vi "AIT 664 - Add Rx Message Port.vi"(0 "Item Ref in":T4 format="%.0x", 5 "Rx Message Port":T1, 11 "error in (no error)":errorcluster) -> (15 "error out":errorcluster)   [LabVIEW 2013, in "AIT 664 Custom Device.lvlib"]
doc: "Add Rx Message Port"
uses:
  AIT 664 Custom Device.lvlib
  <vilib>/NI Veristand/Custom Device API/Custom Device Item Ref.ctl
  Controls/664 - XML Rx Message Port.ctl
  Controls/664 - Sampling Type.ctl
  Controls/664 -Param.ctl
  <vilib>/NI Veristand/Custom Device API/Custom Device Channel.ctl
  <vilib>/NI Veristand/Custom Device API/Custom Device Channel Type.ctl
  Controls and Global/Global.vi
  <vilib>/NI Veristand/Custom Device API/Set Item Property (U32).vi
  <vilib>/NI Veristand/Custom Device API/Set Item Property (Variant).vi
  <vilib>/NI Veristand/Custom Device API/Set Item Property (String).vi
  <vilib>/NI Veristand/Custom Device API/Set Item Property (Boolean).vi
  <vilib>/NI Veristand/Custom Device API/Custom Device API.lvlib
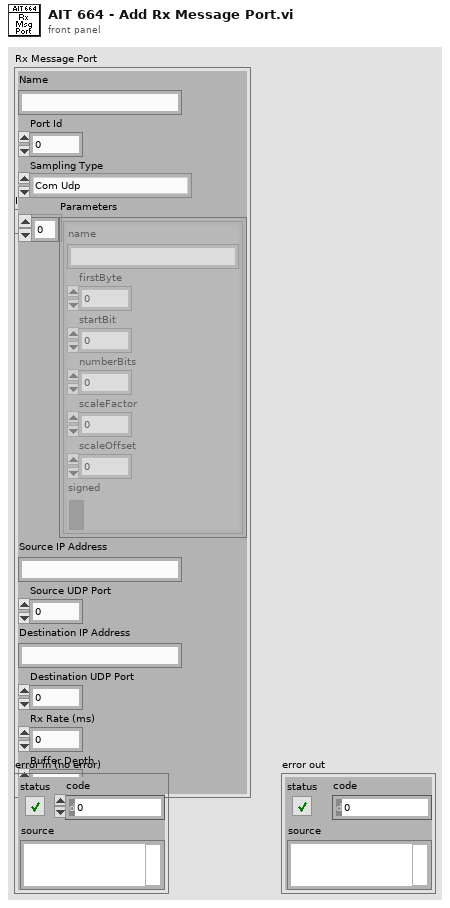
[diagram p1: front panel]
types:
  T1 = typedef "AIT 664 Custom Device.lvlib/664 - XML Rx Message Port.ctl" = cluster{"Name":string, "Port Id":u32, "Sampling Type":T2, "Parameters":T3[], "Source IP Address":string, "Source UDP Port":u32, "Destination IP Address":string, "Destination UDP Port":u32, "Rx Rate (ms)":u32, "Buffer Depth":u32}
  T2 = typedef "AIT 664 Custom Device.lvlib/664 - Sampling Type.ctl" = enum16{"Com Udp", "Com Udp Queuing", "Sap Udp", "Sap Ip", "Sap Mac", "Unknown"}
  T3 = typedef "AIT 664 Custom Device.lvlib/664 -Param.ctl" = cluster{"name":string, "firstByte":i32, "startBit":i32, "numberBits":i32, "scaleFactor":dbl, "scaleOffset":dbl, "signed":bool}
  T4 = typedef "Custom Device API.lvlib/Custom Device Item Ref.ctl" = u64
  T5 = typedef "Custom Device API.lvlib/Custom Device Channel Type.ctl" = enum16{"Input", "Output"}
  T6 = typedef "Custom Device API.lvlib/Custom Device Channel.ctl" = cluster{"Type":T5, "Units":string, "Default Value":dbl, "Faultable":bool, "Scalable":bool}
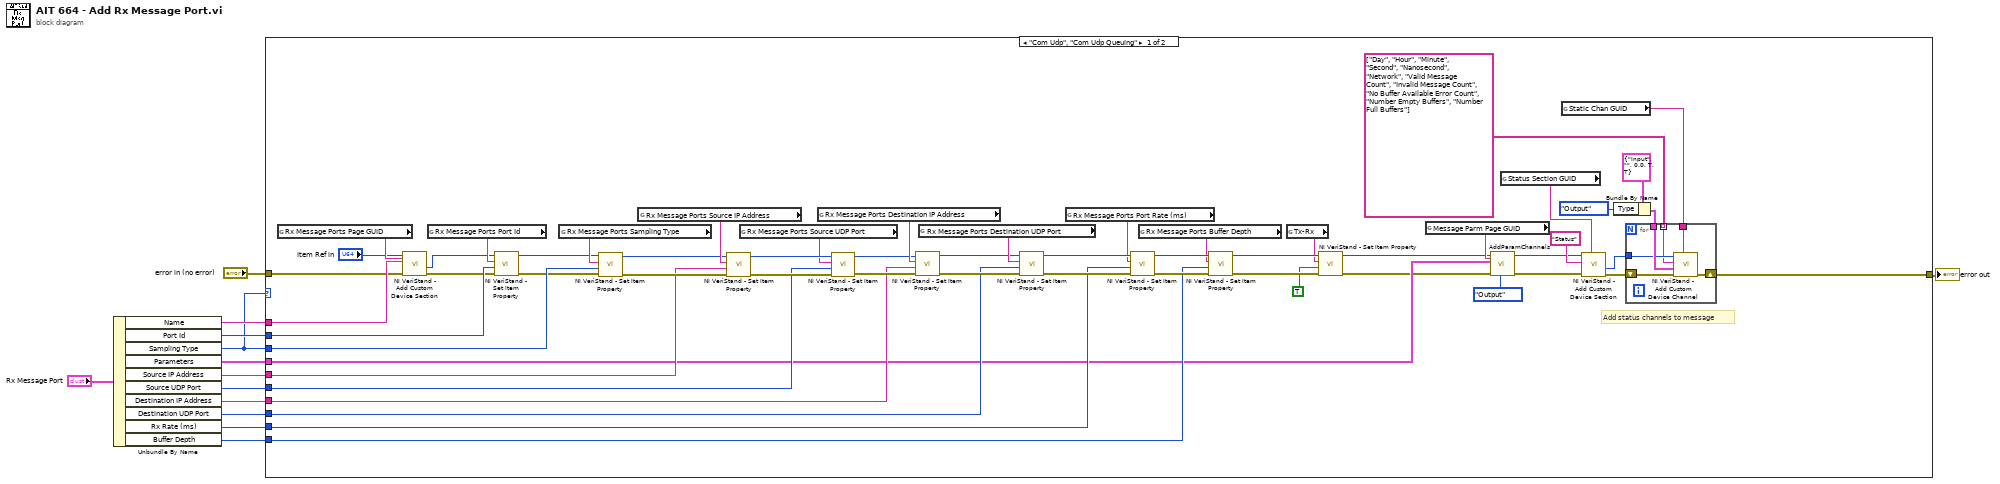
[diagram p0: block diagram]
diagram:
  n1 = Unbundle By Name("Rx Message Port") -> ("Name"=w12:string, "Port Id"=w13:u32, "Sampling Type"=w9:T2, "Parameters"=w10:T3[], "Source IP Address"=w6:string, "Source UDP Port"=w5:u32, "Destination IP Address"=w4:string, "Destination UDP Port"=w3:u32, "Rx Rate (ms)"=w2:u32, "Buffer Depth"=w1:u32)
  n2 = case shown="\"Com Udp\", \"Com Udp Queuing\"" w9 {
    tunnel: w9 -> [w69 _]
    tunnel: w13 -> [w65 _]
    tunnel: w12 -> [w61 _]
    tunnel: w10 -> [w21 _]
    tunnel: "error in (no error)" -> [w48 w77]
    tunnel: [w20 w77] -> w7
    tunnel: w6 -> [w35 _]
    tunnel: w5 -> [w34 _]
    tunnel: w4 -> [w33 _]
    tunnel: w3 -> [w32 _]
    tunnel: w2 -> [w28 _]
    tunnel: w1 -> [w24 _]
    frame "Com Udp", "Com Udp Queuing" {
      # "Add status channels to message"
      n3 = global read "Global.vi" "Rx Message Ports Page GUID"() -> (w62:string)
      n4 = call <vilib>:"NI VeriStand - Add Custom Device Section.vi"("GUID (Default Section)"=w62, "error in (no error)"=w48, "Section Name"=w61, "Parent Ref in"="Item Ref in") -> ("error out"=w63:errorcluster, "Section Ptr"=w64:T4)  [unwired: 4 in, 2 out]
      n5 = global read "Global.vi" "Rx Message Ports Port Id"() -> (w66:string)
      n6 = call-poly <vilib>:"NI VeriStand - Set Item Property.vi"("error in (no error)"=w63, "Value"=w65, "Property Name"=w66, "Item Ref in"=w64) -> ("error out"=w67:errorcluster, "Item Ref out"=w68:T4)  [unwired: 5 in, 1 out]
      n7 = global read "Global.vi" "Rx Message Ports Sampling Type"() -> (w70:string)
      n8 = call-poly <vilib>:"NI VeriStand - Set Item Property.vi"("error in (no error)"=w67, "Value"=w69, "Property Name"=w70, "Item Ref in"=w68) -> ("error out"=w46:errorcluster, "Item Ref out"=w45:T4)  [unwired: 5 in, 1 out]
      n9 = global read "Global.vi" "Rx Message Ports Source IP Address"() -> (w47:string)
      n10 = call-poly <vilib>:"NI VeriStand - Set Item Property.vi"("error in (no error)"=w46, "Value"=w35, "Property Name"=w47, "Item Ref in"=w45) -> ("error out"=w44:errorcluster, "Item Ref out"=w43:T4)  [unwired: 5 in, 1 out]
      n11 = global read "Global.vi" "Rx Message Ports Source UDP Port"() -> (w42:string)
      n12 = global read "Global.vi" "Rx Message Ports Destination IP Address"() -> (w38:string)
      n13 = call-poly <vilib>:"NI VeriStand - Set Item Property.vi"("error in (no error)"=w44, "Value"=w34, "Property Name"=w42, "Item Ref in"=w43) -> ("error out"=w37:errorcluster, "Item Ref out"=w36:T4)  [unwired: 5 in, 1 out]
      n14 = call-poly <vilib>:"NI VeriStand - Set Item Property.vi"("error in (no error)"=w37, "Value"=w33, "Property Name"=w38, "Item Ref in"=w36) -> ("error out"=w39:errorcluster, "Item Ref out"=w40:T4)  [unwired: 5 in, 1 out]
      n15 = global read "Global.vi" "Rx Message Ports Destination UDP Port"() -> (w41:string)
      n16 = call-poly <vilib>:"NI VeriStand - Set Item Property.vi"("error in (no error)"=w39, "Value"=w32, "Property Name"=w41, "Item Ref in"=w40) -> ("error out"=w31:errorcluster, "Item Ref out"=w30:T4)  [unwired: 5 in, 1 out]
      n17 = global read "Global.vi" "Rx Message Ports Port Rate (ms)"() -> (w29:string)
      n18 = call-poly <vilib>:"NI VeriStand - Set Item Property.vi"("error in (no error)"=w31, "Value"=w28, "Property Name"=w29, "Item Ref in"=w30) -> ("error out"=w26:errorcluster, "Item Ref out"=w27:T4)  [unwired: 5 in, 1 out]
      n19 = global read "Global.vi" "Rx Message Ports Buffer Depth"() -> (w25:string)
      n20 = call-poly <vilib>:"NI VeriStand - Set Item Property.vi"("error in (no error)"=w26, "Value"=w24, "Property Name"=w25, "Item Ref in"=w27) -> ("error out"=w19:errorcluster, "Item Ref out"=w17:T4)  [unwired: 5 in, 1 out]
      n21 = global read "Global.vi" "Tx-Rx"() -> (w15:string)
      n22 = call-poly <vilib>:"NI VeriStand - Set Item Property.vi"("error in (no error)"=w19, "Value"=TRUE, "Property Name"=w15, "Item Ref in"=w17) -> ("error out"=w18:errorcluster, "Item Ref out"=w16:T4)  [unwired: 5 in, 1 out]
      n23 = global read "Global.vi" "Message Parm Page GUID"() -> (w50:string)
      n24 = call "AddParamChannels.vi"("Parm Page GUID"=w50, "Type"=Custom_Device_Channel_Type."Output", "error in"=w18, "Parameters to add"=w21, "Node Ref In"=w16) -> ("error out"=w22:errorcluster, "Node Ref Out"=w23:T4)  [unwired: 5 in]
      n25 = global read "Global.vi" "Status Section GUID"() -> (w53:string)
      n26 = global read "Global.vi" "Static Chan GUID"() -> (w54:string)
      n27 = call <vilib>:"NI VeriStand - Add Custom Device Section.vi"("GUID (Default Section)"=w53, "error in (no error)"=w22, "Section Name"="Status", "Parent Ref in"=w23) -> ("error out"=w51:errorcluster, "Section Ptr"=w56:T4)  [unwired: 4 in, 2 out]
      n28 = Bundle By Name(cluster=T6 {"Type"=enum."Input", "Units"="", "Default Value"=0.0, "Faultable"=TRUE, "Scalable"=TRUE} ("Channel"), "Type"=Custom_Device_Channel_Type."Output") -> (w57:T6)
      n29 = for {
        tunnel: w57 -> [w76]
        tunnel: w54 -> [w75]
        tunnel: w56 -> [w74]
        tunnel: string[] ["Day", "Hour", "Minute", "Second", "Nanosecond", "Network", "Valid Message Count", "Invalid Message Count", "No Buffer Available Error Count", "Number Empty Buffers", "Number Full Buffers"] -> [w73] mode=indexing
        shift-right: [w72] -> w20
        shift-left: w51 -> [w71]
        n30 = call <vilib>:"NI VeriStand - Add Custom Device Channel.vi"("GUID (Default Channel)"=w75, "error in (no error)"=w71, "Channel"=w76, "Channel Name"=w73, "Parent Ref in"=w74) -> ("error out"=w72:errorcluster)  [unwired: 3 in, 3 out]
      }
    }
    frame "Sap Udp".."Unknown", Default {
    }
  }
  "error out" <- w7
